vi "AddressEncoder.vi"(1 "Address Cluster":T1={"Subsystem Id"=90, "Node Id"=1, "Component Id"=1}) -> (0 "Address":u32)   [LabVIEW 2009]
uses:
  Address.ctl
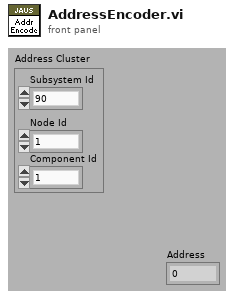
[diagram p1: front panel]
types:
  T1 = typedef "Address.ctl" = cluster{"Subsystem Id":u16, "Node Id":u8, "Component Id":u8}
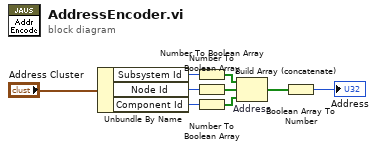
[diagram p0: block diagram]
diagram:
  n1 = Unbundle By Name("Address Cluster") -> ("Subsystem Id"=w6:u16, "Node Id"=w5:u8, "Component Id"=w4:u8)
  n2 = Number To Boolean Array(number=w6) -> (Boolean array=w3:bool[])
  n3 = Number To Boolean Array(number=w5) -> (Boolean array=w8:bool[])
  n4 = Number To Boolean Array(number=w4) -> (Boolean array=w9:bool[])
  n5 = Build Array (concatenate) "Address"(w3, w8, w9) -> (w7:bool[])
  n6 = Boolean Array To Number(Boolean array=w7) -> (number=→"Address":u32)
